vi "Create Multiple Messages.vi"(0 "names":string[](array[string]), 5 "values":string[](array[string]), 7 "attributes":T2[](array[typedef]), 11 "error in":errorcluster, 12 "priority messages (F)":bool, 13 "acknowledge messages (F)":bool) -> (4 "messages":T1[](array[typedef]), 15 "error out":errorcluster)   [LabVIEW 2013, in "AMC.lvlib"]
doc: "Creates an array of AMC messages."
uses:
  AMC.lvlib
  <vilib>/NI/Tools/Keyed Array/KeyedArray.ctl
  Message.ctl
  <vilib>/NI/Tools/Keyed Array/Tools_KeyedArray.lvlib
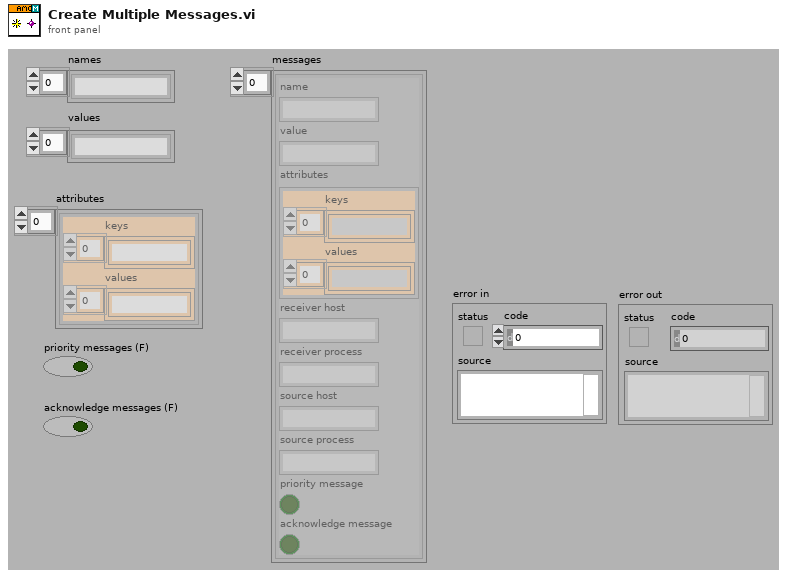
[diagram p1: front panel]
types:
  T1 = typedef "AMC.lvlib/Message.ctl" = cluster{"name":string, "value":string, "attributes":T2, "receiver host":string, "receiver process":string, "source host":string, "source process":string, "priority message":bool, "acknowledge message":bool}
  T2 = typedef "Tools_KeyedArray.lvlib/KeyedArray.ctl" = cluster{"keys":string[], "values":string[]}
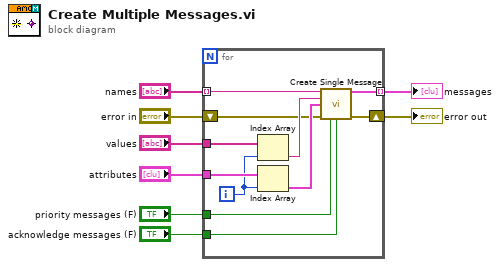
[diagram p0: block diagram]
diagram:
  n1 = for {
    tunnel: "names" -> [w16] mode=indexing
    tunnel: "values" -> [w19]
    tunnel: "attributes" -> [w18]
    tunnel: [w15] -> w5 mode=indexing
    tunnel: "priority messages (F)" -> [w12]
    tunnel: "acknowledge messages (F)" -> [w11]
    shift-right: [w9] -> w1
    shift-left: "error in" -> [w10]
    i -> [w17]
    n2 = Index Array(array=w19, index=w17) -> (element=w14:string)
    n3 = Index Array(array=w18, index=w17) -> (element=w13:T2)
    n4 = call "Create Single Message.vi"("name"=w16, "value"=w14, "attributes"=w13, "error in"=w10, "priority message (F)"=w12, "acknowledge message (F)"=w11) -> ("message"=w15:T1, "error out"=w9:errorcluster)  [unwired: 8 in]
  }
  "messages" <- w5
  "error out" <- w1
